vi "Import Custom Device (In Place).vi"(8 "error in":errorcluster, 10 "path":path, 11 "custom device ref":T1 format="%.0x") -> (0 "error out":errorcluster, 3 "new custom device ref":T1 format="%.0x")   [LabVIEW 2020, in "Communication Bus Template Scripting.lvlib"]
uses:
  <vilib>/NI VeriStand/Custom Device API/Custom Device Item Ref.ctl
  <vilib>/NI/VeriStand Custom Device Serialization/Import in Place.vi
  Communication Bus Template Scripting.lvlib
  <vilib>/NI/VeriStand Custom Device Serialization/Custom Device Serialization.lvlib
  <vilib>/NI VeriStand/Custom Device API/Custom Device API.lvlib
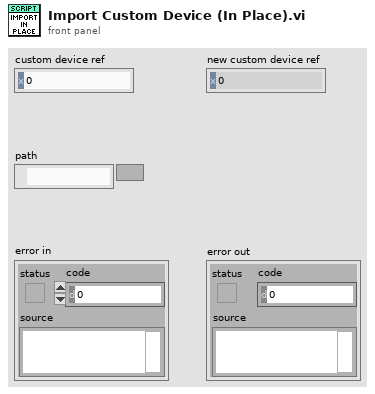
[diagram p1: front panel]
types:
  T1 = typedef "Custom Device API.lvlib/Custom Device Item Ref.ctl" = u64
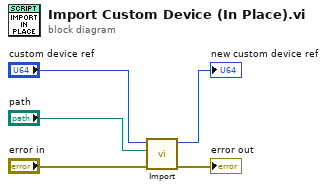
[diagram p0: block diagram]
diagram:
  n1 = call-poly <vilib>:"Import.vi"("error in"="error in", "path"="path", "item ref"="custom device ref") -> ("error out"=→"error out":errorcluster, "new item ref"=→"new custom device ref":T1)  [unwired: 7 in]
